vi "Connect.vi"(8 "error in (no error)":errorcluster caption="entrée d'erreur (pas d'erreur)", 11 "Database Altyor en entrée":refnum<class "Database Altyor Packaging.lvclass">) -> (0 "error out":errorcluster caption="sortie d'erreur", 3 "Database Altyor en sortie":refnum<class "Database Altyor Packaging.lvclass">)   [LabVIEW 2020, in "Library Instrument & Equipement.lvlib" / "Library Database.lvlib" / "Database Altyor Packaging.lvclass"]
uses:
  Database Altyor Packaging.lvclass
  Database drivers/Database Drivers.lvclass
  Database Altyor Packaging.lvclass/Database Altyor Packaging.ctl
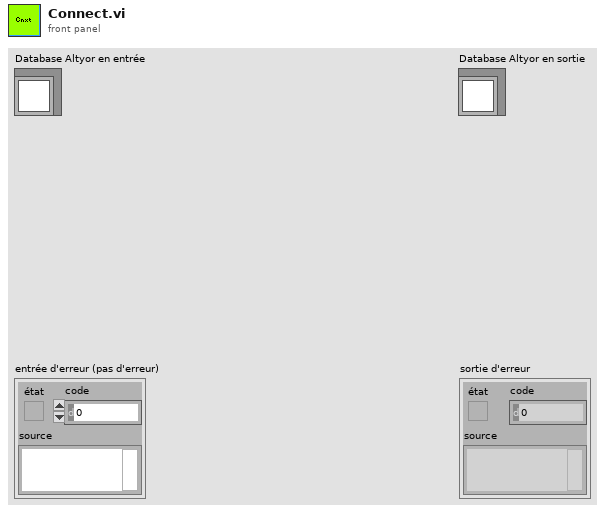
[diagram p1: front panel]
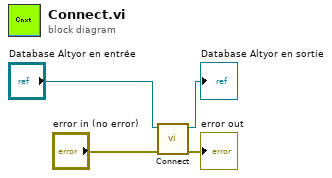
[diagram p0: block diagram]
diagram:
  n1 = call-parent "Connect.vi"("error in (no error)"="error in (no error)", "Database Drivers en entrée"="Database Altyor en entrée") -> ("error out"=→"error out":errorcluster, "Database Drivers en sortie"=→"Database Altyor en sortie":refnum<class "Database Altyor Packaging.lvclass">)  [unwired: 8 in]
